vi "Rectangle0005.vi"   [LabVIEW 2013]
uses:
  <vilib>/Heliosphere Research LLC/Advanced Plotting Toolkit/api_core/NewPlotProperties.ctl
  <vilib>/Heliosphere Research LLC/Advanced Plotting Toolkit/typedefs/PlotColor.ctl
  <vilib>/Heliosphere Research LLC/Advanced Plotting Toolkit/api_core/NewPlotScales.ctl
  <vilib>/Heliosphere Research LLC/Advanced Plotting Toolkit/Advanced Plotting Toolkit.lvlib
types:
  T1 = typedef "Advanced Plotting Toolkit.lvlib/NewPlotScales.ctl" = enum16{"Default", "Linear", "Log", "Symlog"}
  T2 = typedef "Advanced Plotting Toolkit.lvlib/NewPlotProperties.ctl" = cluster{"Background Color":T3, "Axis Background":T3, "Left Margin":dbl, "Right Margin":dbl, "Bottom Margin":dbl, "Top Margin":dbl, "Aspect Ratio":dbl}
  T3 = typedef "Advanced Plotting Toolkit.lvlib/PlotColor.ctl" = u32
  T4 = typedef "Advanced Plotting Toolkit.lvlib/PlotID.ctl" = i32
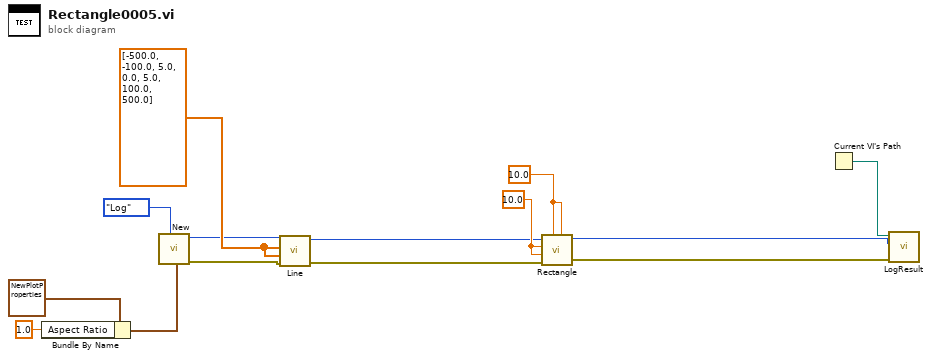
[diagram p0: block diagram]
diagram:
  w7 = dbl[] [-500.0, -100.0, 5.0, 0.0, 5.0, 100.0, 500.0] ("X Data")
  w4 = 10.0 ("Radius")
  w13 = 10.0 ("X Position")
  n1 = Bundle By Name(cluster=T2 {"Background Color"=2147483647, "Axis Background"=2147483647, "Left Margin"=nan, "Right Margin"=nan, "Bottom Margin"=nan, "Top Margin"=nan, "Aspect Ratio"=nan} ("New Plot Properties"), "Aspect Ratio"=1.0) -> (w9:T2)
  n2 = call <vilib>:"New.vi"("Properties"=w9, "X Axis Scale"=NewPlotScales."Log") -> ("error out"=w5:errorcluster, "Plot ID"=w6:T4)  [unwired: 8 in]
  n3 = call <vilib>:"Line.vi"("error in (no error)"=w5, "Y Data"=w7, "X Data"=w7, "Plot ID"=w6) -> ("error out"=w1:errorcluster, "Plot ID out"=w2:T4)  [unwired: 6 in]
  n4 = call <vilib>:"Rectangle.vi"("Height"=w4, "Width"=w4, "error in (no error)"=w1, "Y Position"=w13, "X Position"=w13, "Plot ID"=w2) -> ("error out"=w11:errorcluster, "Plot ID Out"=w12:T4)  [unwired: 4 in]
  n5 = Current VI's Path() -> (path=w14:path)
  n6 = call "LogResult.vi"("Test Result"=w11, "Test Artifact"=w12, "VI Path"=w14) -> ()  [unwired: 9 in]
